vi "oscillate.vi"() -> ()   [LabVIEW 2023]
uses:
  <vilib>/DAQmx/read.llb/DAQmx Read (Digital 1D Bool 1Chan 1Samp).vi
  <vilib>/DAQmx/create/channels.llb/DAQmx Create Channel (DI-Digital Input).vi
  <vilib>/DAQmx/miscellaneous.llb/DAQmx Fill In Error Info.vi
panel:
  out "PerisPump_read":string[](array[string])
  out "PerisPump_write":string[](array[string])
  out "sensor":bool[](array[boolean])
  out "current index":i8
  in  "stop":bool
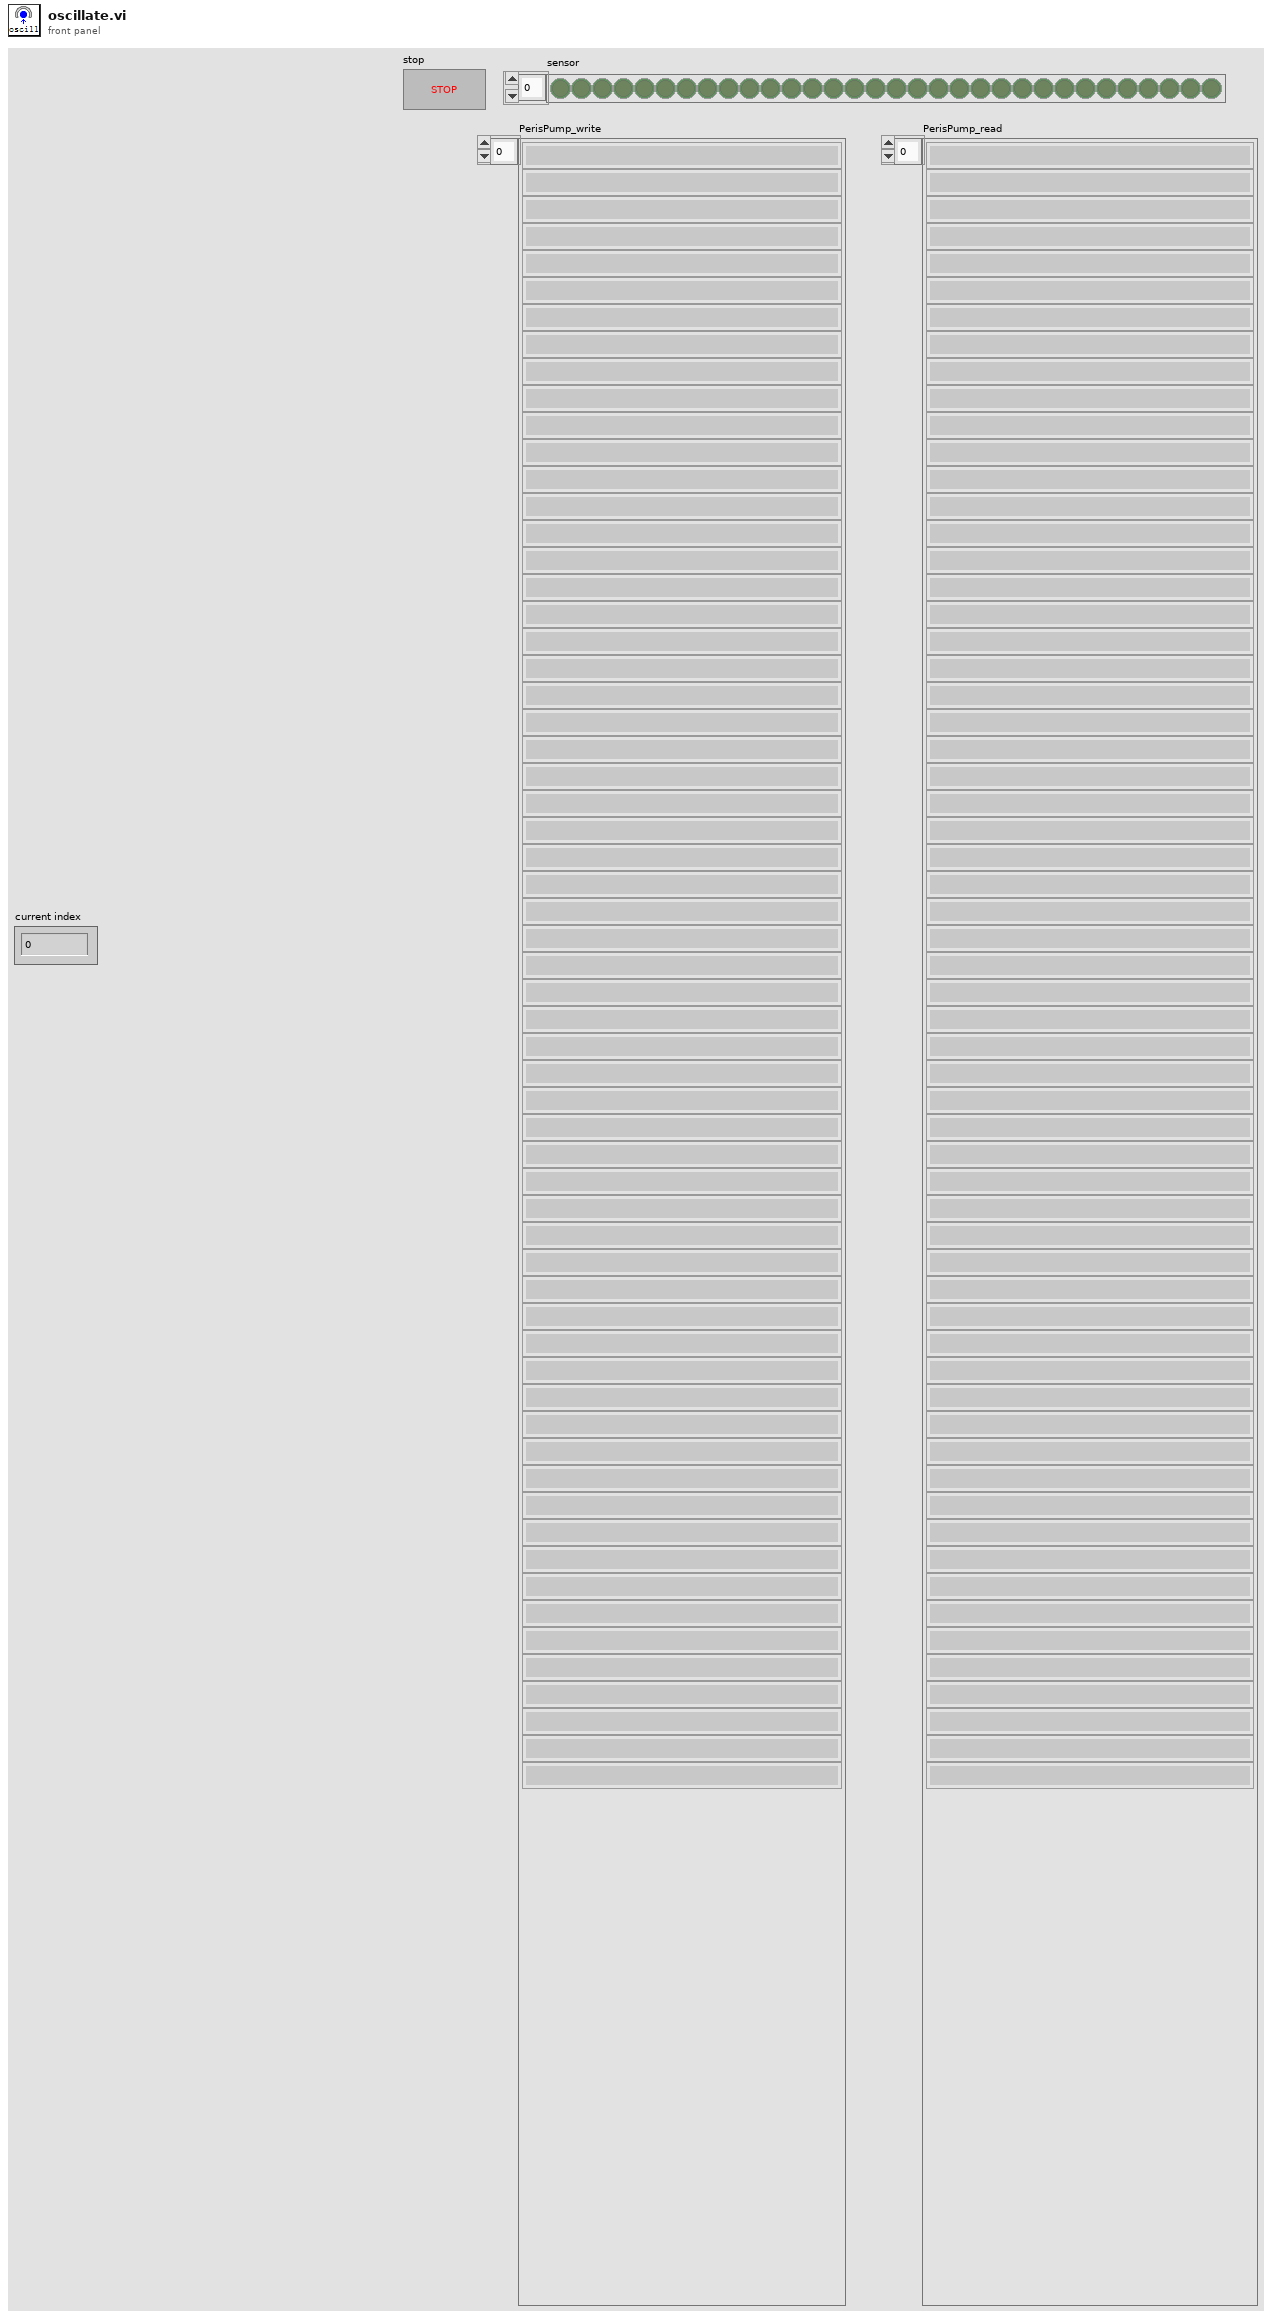
[diagram p1: front panel]
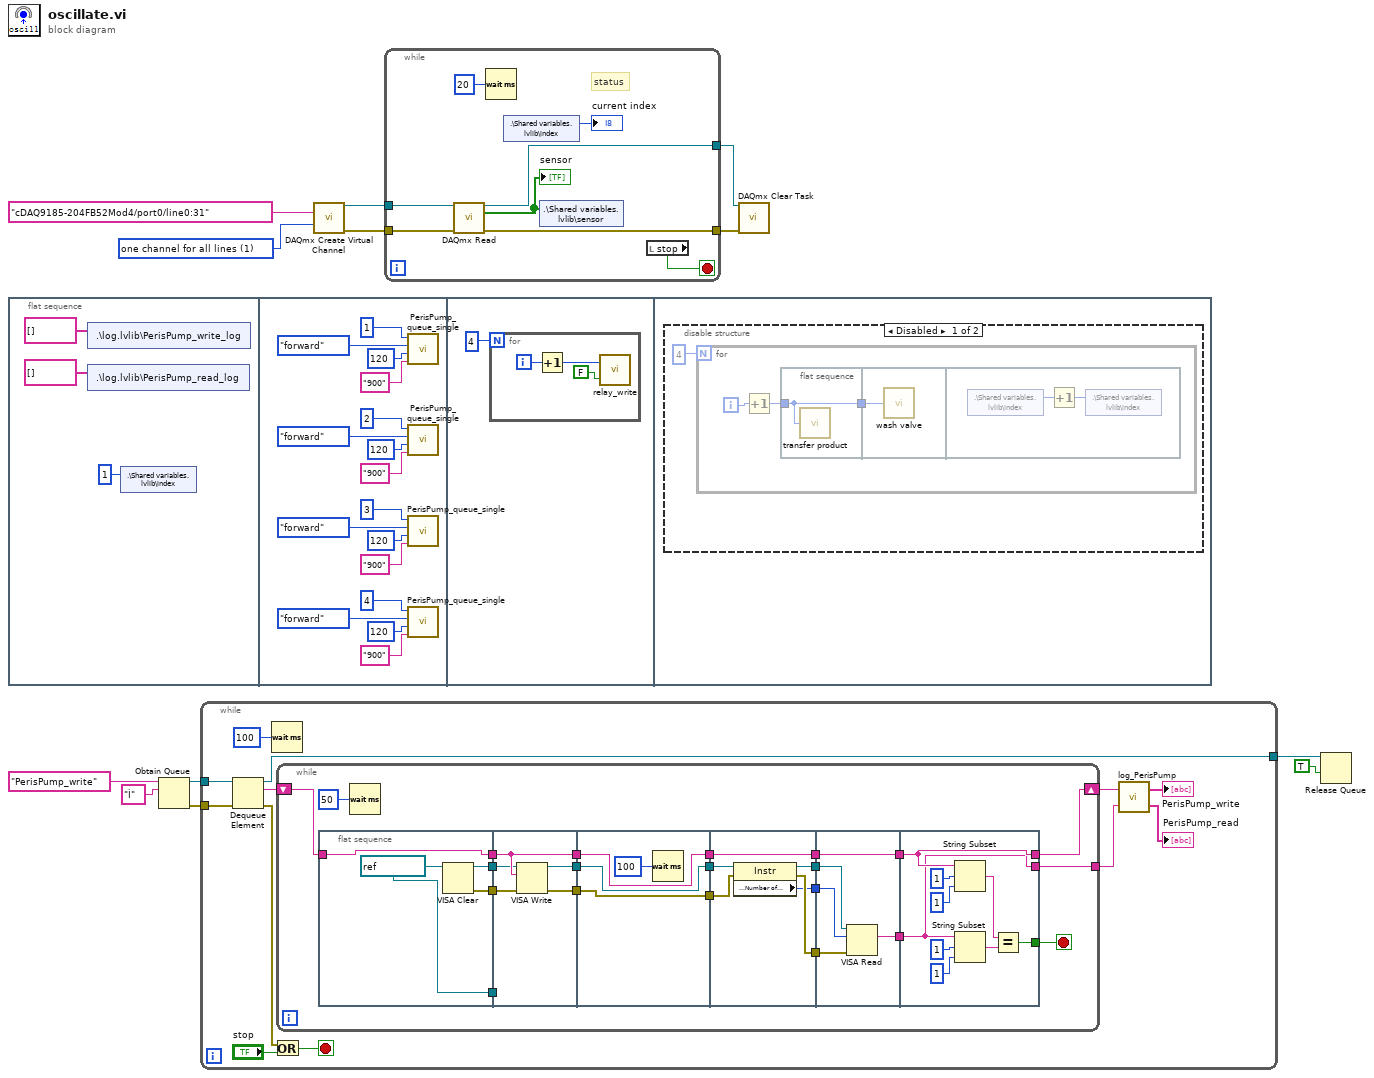
[diagram p0: block diagram]
diagram:
  w5 = 1 items=["one channel for each line", "one channel for all lines"] ("line grouping")
  n1 = flat-sequence {
    frame #0 {
      n2 = shared-variable ".\\log.lvlib\\PerisPump_write_log"(string[] [] ("appended array")) -> ()  [unwired: 1 in, 1 out]
      n3 = shared-variable ".\\log.lvlib\\PerisPump_read_log"(string[] [] ("appended array")) -> ()  [unwired: 1 in, 1 out]
      n4 = shared-variable ".\\Shared variables.lvlib\\index"(i8 1 ("index")) -> ()  [unwired: 1 in, 1 out]
    }
    frame #1 {
      n5 = call "PerisPump_queue_single.vi"("Step"="900", "Time/min"=120 ("Cycle"), "First step"=enum16{"forward", "backward"}."forward", "Address"=u8 1) -> ()  [unwired: 7 in, 1 out]
      n6 = call "PerisPump_queue_single.vi"("Step"="900", "Time/min"=120 ("Cycle"), "First step"=enum16{"forward", "backward"}."forward", "Address"=u8 2) -> ()  [unwired: 7 in, 1 out]
      n7 = call "PerisPump_queue_single.vi"("Step"="900", "Time/min"=120 ("Cycle"), "First step"=enum16{"forward", "backward"}."forward", "Address"=u8 3) -> ()  [unwired: 7 in, 1 out]
      n8 = call "PerisPump_queue_single.vi"("Step"="900", "Time/min"=120 ("Cycle"), "First step"=enum16{"forward", "backward"}."forward", "Address"=u8 4) -> ()  [unwired: 7 in, 1 out]
    }
    frame #2 {
      n9 = for {
        N: 4 -> [_]
        i -> [w35]
        n10 = Increment(x=w35) -> (x+1=w33:i32)
        n11 = call "relay_write.vi"("on/off"=FALSE, "No."=w33) -> ()  [unwired: 1 out]
      }
    }
    frame #3 {
      n12 = disable-structure shown="Disabled" {
        frame Disabled {
          n13 = for {
            N: 4 -> [_]
            i -> [w39]
            n14 = Increment(x=w39) -> (x+1=w38:i32)
            n15 = flat-sequence {
              tunnel: w38 -> [w40]
              tunnel: [w40] -> w37
              tunnel: w37 -> [w41]
              frame #0 {
                n16 = call "transfer product.vi"("channel"=w40) -> ()  [unwired: 1 in]
              }
              frame #1 {
                n17 = call "wash valve.vi"("channel"=w41) -> ()  [unwired: 1 in]
              }
              frame #2 {
                n18 = shared-variable ".\\Shared variables.lvlib\\index"() -> (w42:i8)  [unwired: 1 in, 1 out]
                n19 = Increment(x=w42) -> (x+1=w43:i8)
                n20 = shared-variable ".\\Shared variables.lvlib\\index"(w43) -> ()  [unwired: 1 in, 1 out]
              }
            }
          }
        }
        frame Enabled {
        }
      }
    }
  }
  n21 = Obtain Queue(name (unnamed)="PerisPump_write", element data type="Ì" ("string")) -> (queue out=w8:refnum<queue>, error out=w7:errorcluster)  [unwired: 3 in, 1 out]
  n22 = while {
    tunnel: w8 -> [w52]
    tunnel: w7 -> [w51]
    tunnel: [w50] -> w9
    stop <- w54 stop-if-true
    n23 = Dequeue Element(queue=w52, error in (no error)=w51) -> (queue out=w50:refnum<queue>, element=w48:string, error out=w49:errorcluster)  [unwired: 1 in, 1 out]
    n24 = Wait (ms)(milliseconds to wait=u32 100) -> ()  [unwired: 1 out]
    n25 = Or(x=w49, y="stop") -> (x .or. y?=w54:bool)
    n26 = while {
      tunnel: [w69] -> w47
      shift-right: [w70] -> w46
      shift-left: w48 -> [w68]
      stop <- w67 stop-if-true
      n27 = flat-sequence {
        tunnel: w68 -> [w80]
        tunnel: [w80] -> w60
        tunnel: [w79] -> w59
        tunnel: [w78] -> w58
        tunnel: [w77] -> w57
        tunnel: [w83] -> w66
        tunnel: [w85] -> w64
        tunnel: [w84] -> w62
        tunnel: w60 -> [w83]
        tunnel: w59 -> [_]
        tunnel: w58 -> [w82]
        tunnel: w57 -> [w81]
        tunnel: w66 -> [w89]
        tunnel: [w89] -> w65
        tunnel: w64 -> [w88]
        tunnel: [w88] -> w63
        tunnel: w62 -> [w87]
        tunnel: [w87] -> w61
        tunnel: w65 -> [w95]
        tunnel: w63 -> [w94]
        tunnel: [w95] -> w76
        tunnel: [w93] -> w75
        tunnel: [w92] -> w74
        tunnel: w61 -> [w91]
        tunnel: [w90] -> w73
        tunnel: w76 -> [w100]
        tunnel: w75 -> [w98]
        tunnel: w74 -> [w99]
        tunnel: w73 -> [w96]
        tunnel: [w100] -> w72
        tunnel: [w97] -> w71
        tunnel: [w104] -> w69
        tunnel: [w107] -> w70
        tunnel: w72 -> [w107]
        tunnel: w71 -> [w104]
        tunnel: [w101] -> w67
        frame #0 {
          w79 = refnum<visa-resource-name> "COM3" ("VISA resource name")
          n28 = VISA Clear(VISA resource name=w79) -> (VISA resource name out=w78:refnum<visa-resource-name>, error out=w77:errorcluster)  [unwired: 1 in]
        }
        frame #1 {
          n29 = VISA Write(VISA resource name=w82, write buffer=w83, error in (no error)=w81) -> (VISA resource name out=w85:refnum<visa-resource-name>, error out=w84:errorcluster)  [unwired: 1 out]
        }
        frame #2 {
          n30 = Wait (ms)(milliseconds to wait=u32 100) -> ()  [unwired: 1 out]
        }
        frame #3 {
          n31 = property class="Instr"(reference=w94, error in=w91) -> (reference out=w93:refnum<visa-resource-name>, error out=w92:errorcluster, "Serial Settings:Number of Bytes at Serial Port"=w90:u32)
        }
        frame #4 {
          n32 = VISA Read(VISA resource name=w98, byte count=w96, error in (no error)=w99) -> (read buffer=w97:string)  [unwired: 3 out]
        }
        frame #5 {
          n33 = String Subset(string=w107, offset (0)=1, length (rest)=1 ("length (rest)")) -> (substring=w102:string)
          n34 = String Subset(string=w104, offset (0)=1, length (rest)=1 ("length (rest)")) -> (substring=w103:string)
          n35 = Equal?(x=w102, y=w103) -> (x = y?=w101:bool)
        }
      }
      n36 = Wait (ms)(milliseconds to wait=u32 50) -> ()  [unwired: 1 out]
    }
    n37 = call "log_PerisPump.vi"("read string"=w47, "write string"=w46) -> ("PerisPump_read"=→"PerisPump_read":string[], "PerisPump_write"=→"PerisPump_write":string[])
  }
  n38 = call-poly <vilib>:"DAQmx Create Virtual Channel.vi"("lines"=tag "cDAQ9185-204FB52Mod4/port0/line0:31", "line grouping"=w5) -> ("task out"=w4:refnum<k21>, "error out"=w3:errorcluster)  [unwired: 12 in]
  n39 = while {
    tunnel: w4 -> [w114]
    tunnel: w3 -> [w113]
    tunnel: [w111] -> w2
    tunnel: [w110] -> w1
    stop <- w115 stop-if-true
    # "status"
    n40 = call-poly <vilib>:"DAQmx Read.vi"("task/channels in"=w114, "error in"=w113) -> ("task out"=w111:refnum<k21>, "data"=w112:bool[], "error out"=w110:errorcluster)  [unwired: 11 in]
    "sensor" <- w112
    n41 = Wait (ms)(milliseconds to wait=u32 20) -> ()  [unwired: 1 out]
    n42 = shared-variable ".\\Shared variables.lvlib\\index"() -> (→"current index":i8)  [unwired: 1 in, 1 out]
    n43 = shared-variable ".\\Shared variables.lvlib\\sensor"(w112) -> ()  [unwired: 1 in, 1 out]
    n44 = local read "stop"() -> (w115:bool)
  }
  n45 = call <vilib>:"DAQmx Clear Task.vi"("task in"=w2, "error in"=w1) -> ()  [unwired: 13 in, 1 out]
  n46 = Release Queue(queue=w9, force destroy? (F)=TRUE) -> ()  [unwired: 1 in, 3 out]
